vi "OFBS_readTestData.vi"(8 "error in (no error)":errorcluster, 9 "ControlRefs":T1, 10 "NumberOfChannels":i32, 11 "OFBS class in":refnum<class "OptFreqBandsSearch.lvclass">) -> (0 "error out":errorcluster, 3 "OFBS class out":refnum<class "OptFreqBandsSearch.lvclass">)   [LabVIEW 2016, in "Optimal Frequency Bands Search.lvlib" / "OptFreqBandsSearch.lvclass"]
doc: "Метод, реализующий чтение тестовых данных (проб) из xml файла и меток класов из txt файла"
uses:
  OptFreqBandsSearch.lvclass
  OptFreqBandsSearch.lvclass/OptFreqBandsSearch.ctl
  <vilib>/Utility/file.llb/Read From Spreadsheet File (string).vi
  <vilib>/xml/Load XML File.vi
  <vilib>/xml/Close Reference(Node).vi
  _XML_EEG_Features/XML_EEG_Features.lvlib
  <vilib>/xml/NI_XML.lvlib
panel:
  # "This VI is a part of BCI Design library, http://www.ru-bci.org \nCopyright © 2020, Sotnikov Peter, All rights reserved. License: CC BY-NC 4.0"
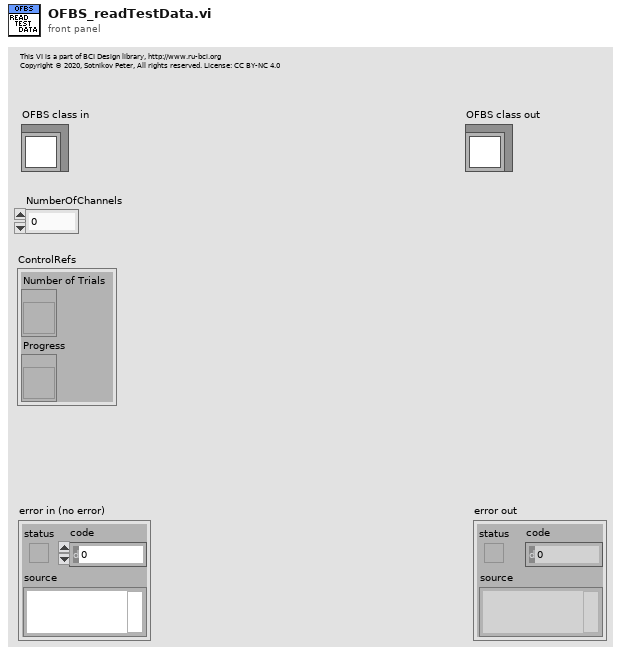
[diagram p1: front panel]
types:
  T1 = cluster{"Number of Trials":refnum<vi>, "Progress":refnum<vi>}
  T2 = typedef "XML_EEG_Features.lvlib/XML_FF_Header.ctl" = cluster{"NumberOfTrials":i32, "NumberOfClasses":i32, "FeatureVectorLength":i32, "FeatureExtractionMethod":string}
  T3 = typedef "XML_EEG_Features.lvlib/XML_FF_Trial.ctl" = cluster{"ClassLabel":string, "FeatureVector":dbl[]}
  T4 = cluster{"String":string, "FeatureVector":dbl[][]}
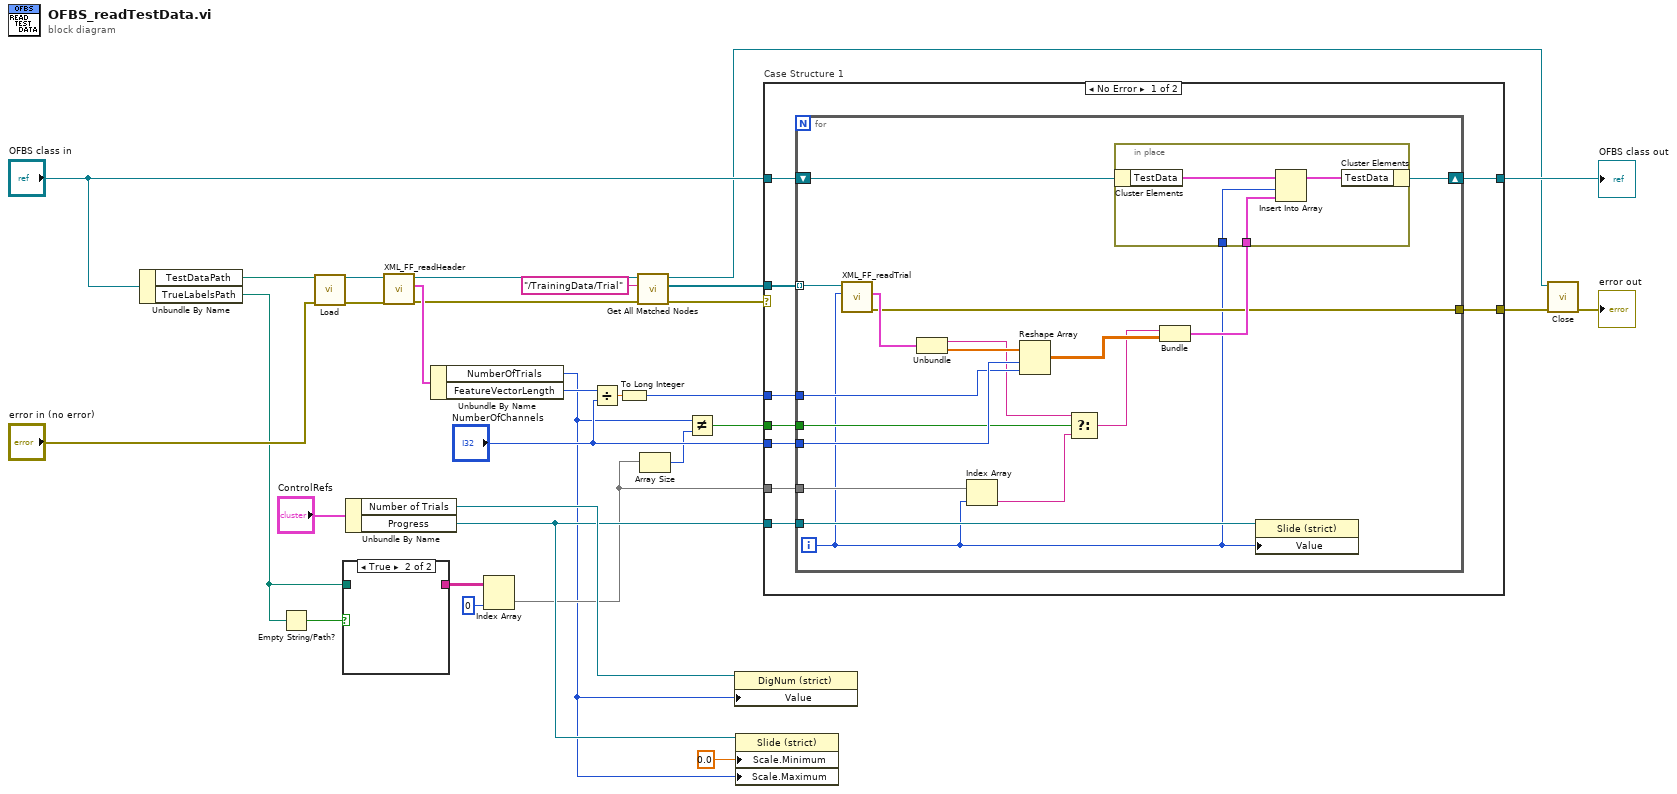
[diagram p0: block diagram]
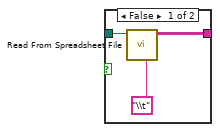
[diagram p2: hidden frame]
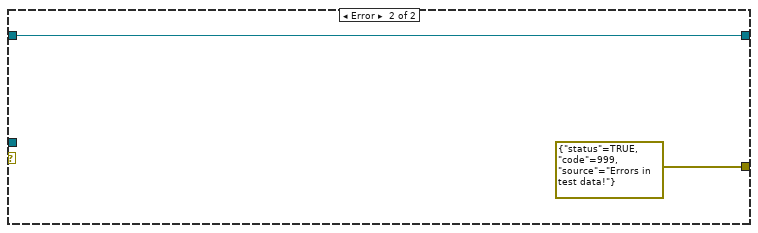
[diagram p3: hidden frame]
diagram:
  n1 = Unbundle By Name("OFBS class in") -> ("TestDataPath"=w31:path, "TrueLabelsPath"=w7:path)
  n2 = Empty String/Path?(string/path=w7) -> (empty?=w8:bool)
  n3 = call-poly <vilib>:"Load.vi"("path to XML document"=w31, "error in (no error)"="error in (no error)") -> ("DOM document out"=w28:refnum<k20>, "error out"=w29:errorcluster)  [unwired: 11 in, 1 out]
  n4 = case shown="True" w8 {
    tunnel: [w33 _] -> w14
    tunnel: w7 -> [w32 _]
    frame False {
      n5 = call-poly <vilib>:"Read From Spreadsheet File.vi"("delimiter (\\t)"="\\t" ("delimiter (\\t)"), "file path (dialog if empty)"=w32) -> ("all rows"=w33:string[][])  [unwired: 5 in, 4 out]
    }
    frame True {
    }
  }
  n6 = Unbundle By Name("ControlRefs") -> ("Number of Trials"=w17:refnum<vi>, "Progress"=w15:refnum<vi>)
  n7 = call "XML_FF_readHeader.vi"("error in (no error)"=w29, "DOM document in"=w28) -> ("error out"=w2:errorcluster, "FF_Header out"=w27:T2, "DOM document out"=w6:refnum<k20>)  [unwired: 7 in]
  n8 = Unbundle By Name(w27) -> ("NumberOfTrials"=w11:i32, "FeatureVectorLength"=w25:i32)
  n9 = Index Array(array=w14, index (col)=0 ("disabled index (col)")) -> (element=w12:string[])  [unwired: 1 in]
  n10 = Divide(x=w25, y="NumberOfChannels") -> (x/y=w20:dbl)
  n11 = To Long Integer(number=w20) -> (32bit integer=w19:i32)
  n12 = call <vilib>:"Get All Matched Nodes.vi"("error in (no error)"=w2, "XPath expression"="/TrainingData/Trial", "node in"=w6) -> ("error out"=w3:errorcluster, "node result array"=w4:refnum<k20>[], "node out"=w5:refnum<k20>)  [unwired: 6 in]
  n13 = Array Size(array=w12) -> (size(s)=w10:i32)
  n14 = Not Equal?(x=w11, y=w10) -> (x != y?=w9:bool)
  n15 = property class="DigNum (strict)"(reference=w17, "Value"=w11) -> ()  [unwired: 1 in, 2 out]
  n16 = property class="Slide (strict)"(reference=w15, "Scale.Minimum"=0.0 ("Data Entry Limits:Minimum"), "Scale.Maximum"=w11) -> ()  [unwired: 1 in, 2 out]
  n17 = case "Case Structure 1" shown="No Error" w3 {
    tunnel: "OFBS class in" -> [w43 w66]
    tunnel: "NumberOfChannels" -> [w42 _]
    tunnel: w19 -> [w41 _]
    tunnel: [w40 w66] -> w23
    tunnel: [w39 errorcluster {"status"=TRUE, "code"=999, "source"="Errors in test data!"} ("error constant")] -> w22
    tunnel: w15 -> [w38 _]
    tunnel: w12 -> [w37 _]
    tunnel: w9 -> [w36 _]
    tunnel: w4 -> [w35 _]
    frame No Error {
      n18 = for {
        shift-right: [w59] -> w40
        shift-left: w43 -> [w60]
        tunnel: w42 -> [w56]
        tunnel: w41 -> [w55]
        tunnel: [w52] -> w39
        tunnel: w38 -> [w51]
        tunnel: w37 -> [w48]
        tunnel: w36 -> [w50]
        tunnel: w35 -> [w44] mode=indexing
        i -> [w47]
        n19 = call "XML_FF_readTrial.vi"("Trial Number"=w47, "DOM document in"=w44) -> ("error out"=w52:errorcluster, "Trial out"=w58:T3)  [unwired: 7 in, 1 out]
        n20 = Unbundle(w58) -> ("ClassLabel"=w49:string, "FeatureVector"=w57:dbl[])
        n21 = Index Array(array=w48, index=w47) -> (element=w46:string)
        n22 = Reshape Array "Reshape Array"(w57, w56, w55) -> (w54:dbl[][])
        n23 = Select(t=w49, s=w50, f=w46) -> (s? t:f=w45:string)
        n24 = Bundle("String"=w45, "FeatureVector"=w54) -> (w53:T4)  [unwired: 1 in]
        n25 = in-place "In Place Element Structure" {
          in-place-border: w53 -> [w62]
          in-place-border: w47 -> [w61]
          n26 = in-place-cluster #1(w60) -> ("TestData"=w64:cluster{"ClassLabel":string, "Trial":dbl[][]}[])
          n27 = Insert Into Array(array=w64, index=w61, new element=w62) -> (w63:cluster{"ClassLabel":string, "Trial":dbl[][]}[])
          n28 = in-place-cluster #1("TestData"=w63) -> (w59:refnum<class "OptFreqBandsSearch.lvclass">)
        }
        n29 = property class="Slide (strict)"(reference=w51, "Value"=w47) -> ()  [unwired: 1 in, 2 out]
      }
    }
    frame Error {
    }
  }
  "OFBS class out" <- w23
  n30 = call-poly <vilib>:"Close.vi"("error in (no error)"=w22, "node"=w5) -> ("error out"=→"error out":errorcluster)  [unwired: 7 in]
